vi "BuildHWI.vi"(8 "error in (no error)":errorcluster, 10 "Master Device in":refnum<class "Master Device.lvclass">, 11 "Novatech in":refnum<class "Novatech.lvclass">) -> (0 "error out":errorcluster, 2 "Master Device out":refnum<class "Master Device.lvclass">, 3 "Novatech out":refnum<class "Novatech.lvclass">)   [LabVIEW 2013, in "Novatech.lvclass"]
doc: "The previous subVI Prune.vi took the \"prepared\" private data and removed unnecessary points. Here in BuildHWI, one should turn the \"prepared\" data into a HWI that can be programmed to the physical device.\n (1) Flatten the data structure and put in normal time order"
uses:
  Novatech.lvclass
  Device/Device.lvclass
  Master Device/Master Device.lvclass
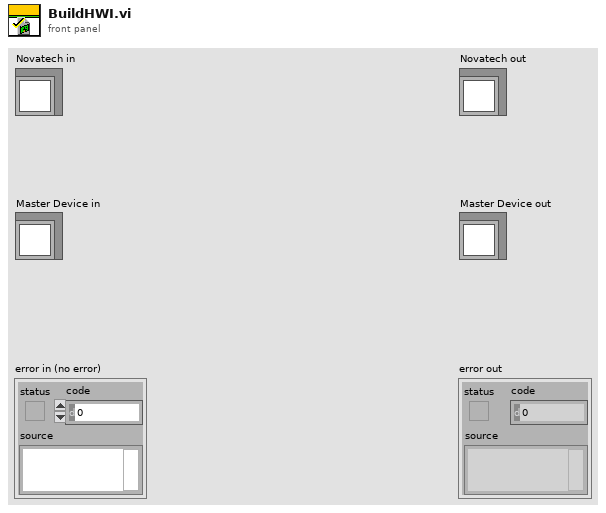
[diagram p1: front panel]
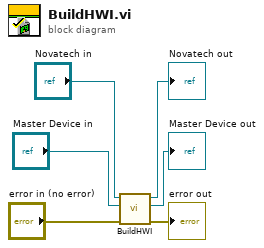
[diagram p0: block diagram]
diagram:
  n1 = call-parent "BuildHWI.vi"("error in (no error)"="error in (no error)", "Master Device in"="Master Device in", "Device in"="Novatech in") -> ("error out"=→"error out":errorcluster, "Master Device out"=→"Master Device out":refnum<class "Master Device.lvclass">, "Device out"=→"Novatech out":refnum<class "Novatech.lvclass">)  [unwired: 6 in]
